vi "DestoryNew.vi"(6 "Stop Traverse":bool, 8 "error in (no error)":errorcluster caption="错误输入（无错误）", 11 "PanelRootNode 输入":refnum<class "PanelRootNode.lvclass"> caption="DNL_LabVIEW Object in") -> (0 "error out":errorcluster caption="错误输出", 3 "PanelRootNode 输出":refnum<class "PanelRootNode.lvclass"> caption="DNL_LabVIEW Object out", 4 "Stop Traverse out":bool)   [LabVIEW 2013, in "PanelRootNode.lvclass"]
uses:
  PanelRootNode.lvclass
  PanelLinkNode/PanelLinkNode.lvclass/PanelLinkNode.ctl
  PanelObject/PanelObject.lvclass
  PanelLinkNode/PanelLinkNode.lvclass
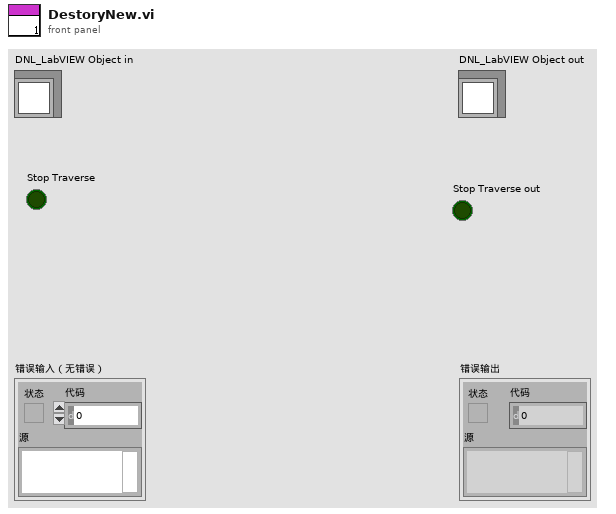
[diagram p1: front panel]
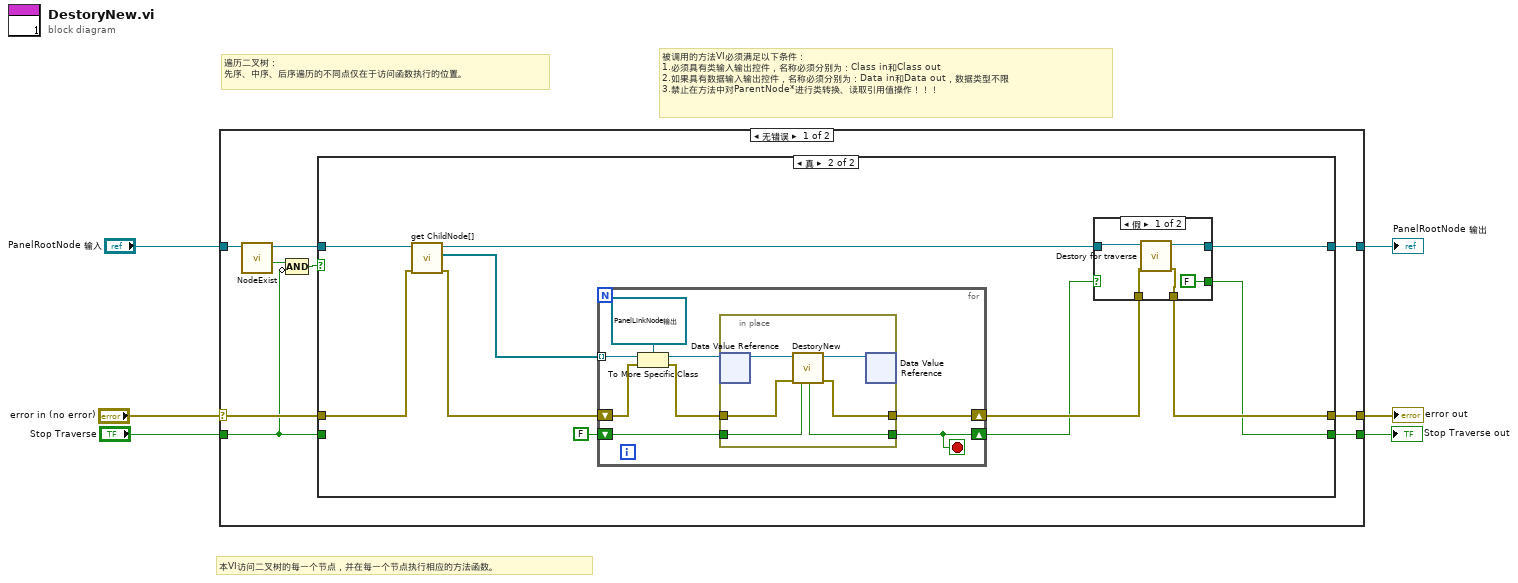
[diagram p0: block diagram]
diagram:
  # "遍历二叉树：\n先序、中序、后序遍历的不同点仅在于访问函数执行的位置。"
  # "本VI访问二叉树的每一个节点，并在每一个节点执行相应的方法函数。"
  # "被调用的方法VI必须满足以下条件：\n1.必须具有类输入输出控件，名称必须分别为：Class in和Class out\n2.如果具有数据输入输出控件，名称必须分别为：Data in和Data out，数据类型不限\n3.禁止在方法中对ParentNode*进行类转换、读取引用值操作！！！"
  n1 = case shown="无错误" "error in (no error)" {
    selector: "error in (no error)" -> [w9 w54]
    tunnel: [w12 w54] -> w2
    tunnel: [w15 w53] -> w3
    tunnel: "PanelRootNode 输入" -> [w14 w53]
    tunnel: "Stop Traverse" -> [w7 w52]
    tunnel: [w8 w52] -> w5
    frame No Error {
      n2 = call-dynamic "NodeExist.vi"("PanelLinkNode 输入"=w14) -> ("Node Exist?"=w11:bool, "PanelLinkNode 输出"=w13:refnum<class "PanelRootNode.lvclass">)  [unwired: 8 in, 1 out]
      n3 = Compound Arithmetic op=AND(w11, invert w7) -> (w10:bool)
      n4 = case shown="真" w10 {
        tunnel: [w18 w29] -> w15
        tunnel: w13 -> [w18 w23]
        tunnel: [w17 w27] -> w12
        tunnel: w9 -> [w17 w21]
        tunnel: [w16 w25] -> w8
        tunnel: w7 -> [w16 _]
        frame False {
        }
        frame True {
          n5 = call "get ChildNode[].vi"("error in (no error)"=w21, "PanelLinkNode输入"=w23) -> ("error out"=w20:errorcluster, "ChildNode*[]"=w22:refnum<data-value>[], "PanelLinkNode输出"=w19:refnum<class "PanelRootNode.lvclass">)  [unwired: 7 in]
          n6 = for {
            tunnel: w22 -> [w45] mode=indexing
            shift-right: [w40] -> w28
            shift-left: w20 -> [w42]
            shift-right: [w39] -> w26
            shift-left: FALSE ("Stop Traverse out") -> [w41]
            stop <- w39 stop-if-true
            n7 = To More Specific Class(target class=refnum<data-value> refnum ("数据值引用"), reference=w45, error in=w42) -> (specific class reference=w44:refnum<data-value>, error out=w43:errorcluster)
            n8 = in-place {
              in-place-border: w43 -> [w49]
              in-place-border: w41 -> [w47]
              in-place-border: [w48] -> w40
              in-place-border: [w46] -> w39
              n9 = in-place-dvr #1(w44) -> (w51:refnum<class "PanelRootNode.lvclass">)  [unwired: 1 out]
              n10 = call-dynamic "DestoryNew.vi"("Stop Traverse"=w47, "error in (no error)"=w49, "PanelRootNode 输入"=w51) -> ("error out"=w48:errorcluster, "PanelRootNode 输出"=w50:refnum<class "PanelRootNode.lvclass">, "Stop Traverse out"=w46:bool)  [unwired: 6 in]
              n11 = in-place-dvr #1(w50) -> ()  [unwired: 2 out]
            }
          }
          n12 = case shown="假" w26 {
            selector: w26 -> [_ w35]
            tunnel: [w33 w37] -> w29
            tunnel: w28 -> [w32 w36]
            tunnel: [w31 w36] -> w27
            tunnel: w19 -> [w34 w37]
            tunnel: [FALSE w35] -> w25
            frame False {
              n13 = call "Destory for traverse.vi"("error in (no error)"=w32, "Class in"=w34) -> ("error out"=w31:errorcluster, "Class out"=w33:refnum<class "PanelRootNode.lvclass">)  [unwired: 8 in]
            }
            frame True {
            }
          }
        }
      }
    }
    frame Error {
    }
  }
  "error out" <- w2
  "PanelRootNode 输出" <- w3
  "Stop Traverse out" <- w5
